vi "Teleop.vi"(10 "Match Info":T1={"Autonomous Elapsed Seconds"=0.0, "TeleOp Elapsed Seconds"=0.0, "Disabled Elapsed Seconds"=0.0, "Visited Autonomous"=FALSE, "Visited TeleOp"=FALSE, "Visited Disabled"=FALSE, "Autonomous Settings"={"Autonomous Style"=enum."Independent", "VI Refnum"=refnum}}, 11 "Call Context":T2) -> ()   [LabVIEW 2019]
doc: "This VI is called for each TeleOp packet received from the DS where the robot is not disabled. It is often used to read from the joysticks and update I/O or to update setpoints for timed control loops. It should complete and return within 20 milliseconds or it may miss DS packets."
uses:
  <vilib>/Rock Robotics/WPI/DriverStation/WPI_DriverStationDerivedRobotMode.ctl
  <vilib>/Rock Robotics/WPI/DriverStation/WPI_DriverStationMatch Info.ctl
  <vilib>/Rock Robotics/WPI/ThirdParty/JAS_Junk/TrajLib/Conv_Meters_Feet.vi
  <vilib>/Rock Robotics/WPI/ThirdParty/JAS_Junk/TrajLib/Conv_Radians_Deg.vi
  <vilib>/Rock Robotics/WPI/Utilities/WPI_GetSetVariantRefNum.vi
  <vilib>/Rock Robotics/Network Tables/NT Write Boolean Array.vi
  <vilib>/Rock Robotics/Network Tables/NT Write Numeric Array.vi
  <vilib>/Rock Robotics/WPI/Joystick/WPI_JoystickArcadeMapping.vi
  Robot Global Data.vi
  <vilib>/Rock Robotics/Network Tables/NT Read Boolean.vi
  <vilib>/Rock Robotics/WPI/ThirdParty/JAS_Junk/TrajLib/Trajectory_Library.lvlib
  <vilib>/Rock Robotics/Network Tables/NT Read Number.vi
panel:
  out "Sample Slider 0":dbl(slide) scale=0.0..5.0
  out "Sample Boolean 1":bool
  out "Sample Boolean 0":bool
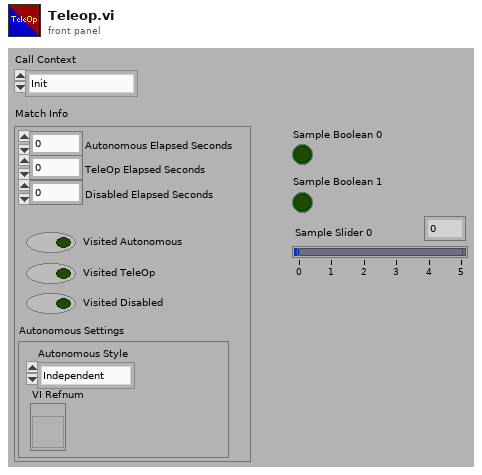
[diagram p1: front panel]
types:
  T1 = typedef "WPI_DriverStationMatch Info.ctl" = cluster{"Autonomous Elapsed Seconds":dbl, "TeleOp Elapsed Seconds":dbl, "Disabled Elapsed Seconds":dbl, "Visited Autonomous":bool, "Visited TeleOp":bool, "Visited Disabled":bool, "Autonomous Settings":cluster{"Autonomous Style":enum16{"Iterative", "Independent"}, "VI Refnum":refnum<vi>}}
  T2 = typedef "WPI_DriverStationDerivedRobotMode.ctl" = enum16{"Init", "Execute", "Stop"}
  T3 = typedef "WPI_JoystickDevRef.ctl" = cluster{"Device":T4}
  T4 = typedef "WPI_JoystickDeviceEnum.ctl" = enum16{"USB 0", "USB 1", "USB 2", "USB 3", "USB 4", "USB 5"}
  T5 = typedef "Trajectory_Library.lvlib/RAMSETE.ctl" = cluster{"B":dbl, "Zeta":dbl, "poseTolerance":T6, "poseError":T6, "Enabled":bool}
  T6 = typedef "Trajectory_Library.lvlib/POSE2D.ctl" = cluster{"TRANSLATION":T7, "ROTATION":T8}
  T7 = typedef "Trajectory_Library.lvlib/TRANSLATION2D.ctl" = cluster{"X":dbl, "Y":dbl}
  T8 = typedef "Trajectory_Library.lvlib/ROTATION2D.ctl" = cluster{"VALUE":dbl, "COS":dbl, "SIN":dbl}
  T9 = typedef "Trajectory_Library.lvlib/TRAJ_STATE.ctl" = cluster{"TimeSeconds":dbl, "Velocity":dbl, "Acceleration":dbl, "POSE":T6, "Curvature":dbl}
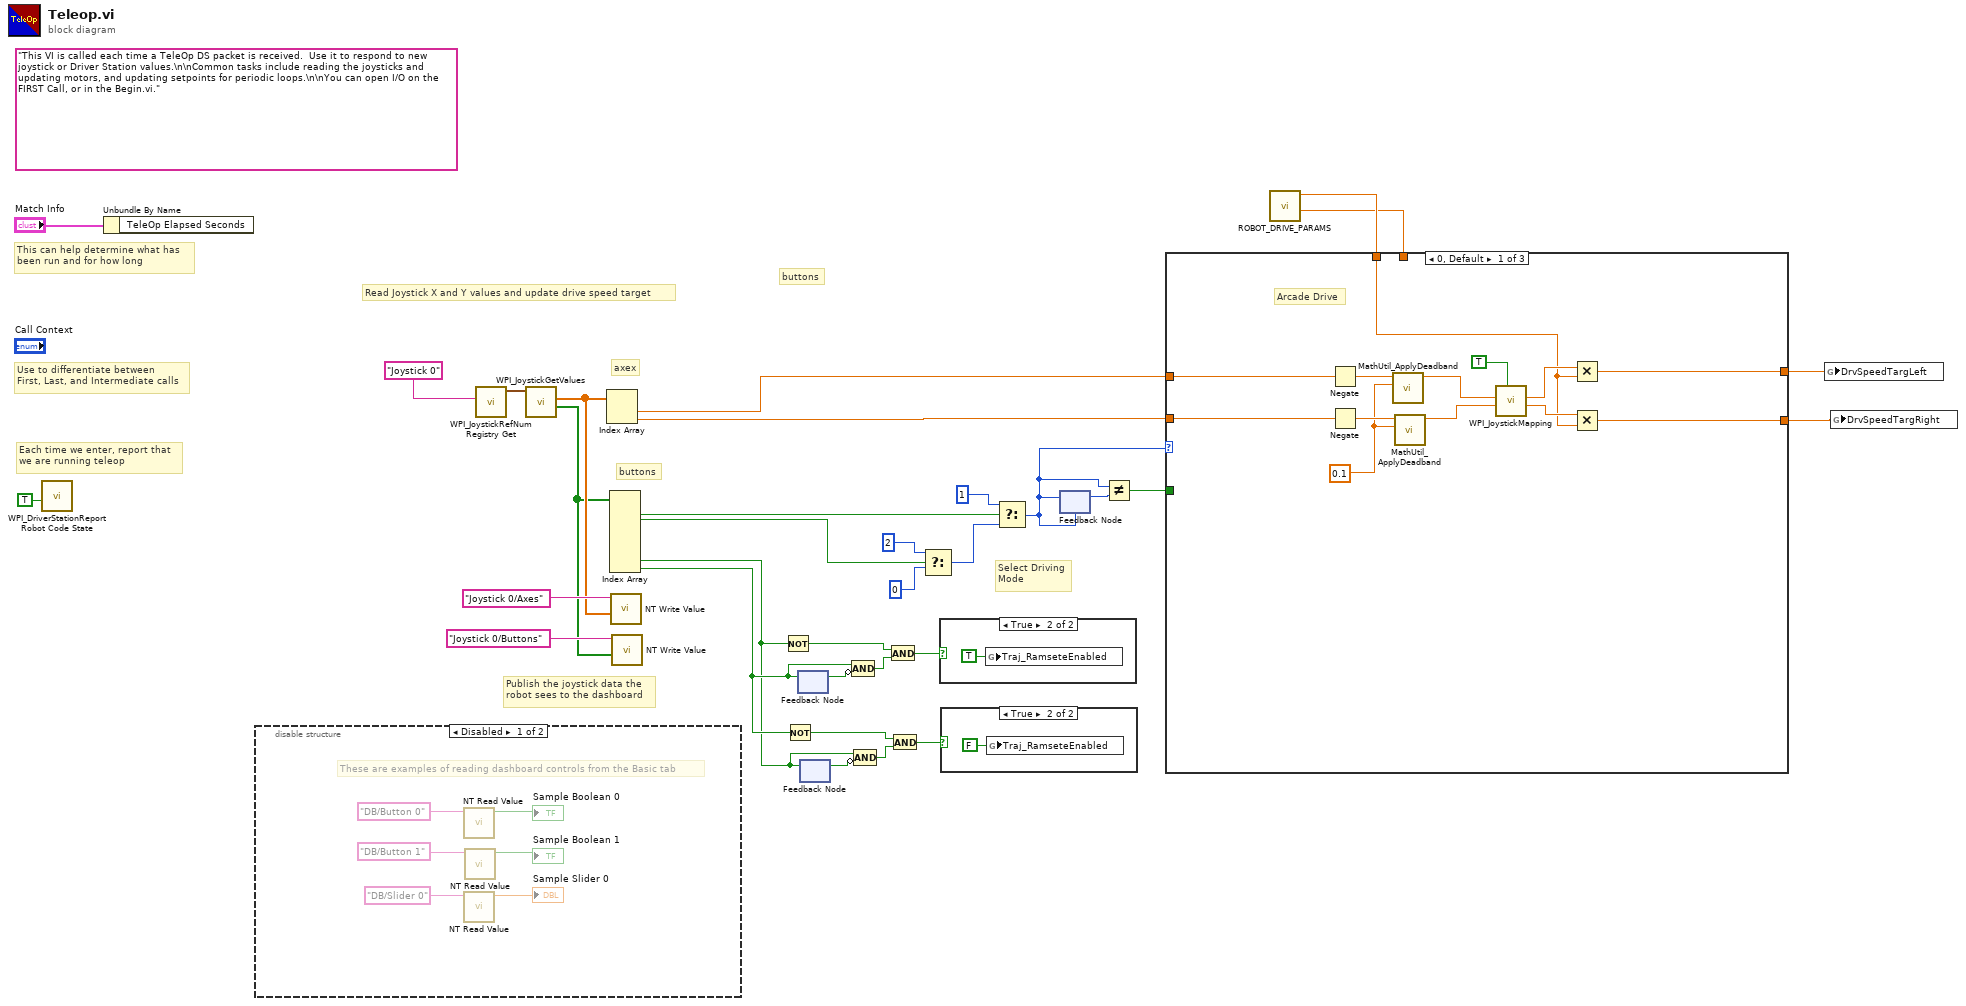
[diagram p0: block diagram]
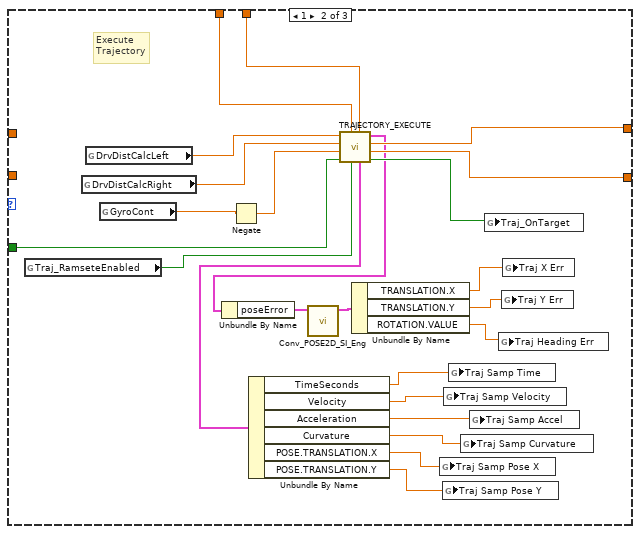
[diagram p4: hidden frame]
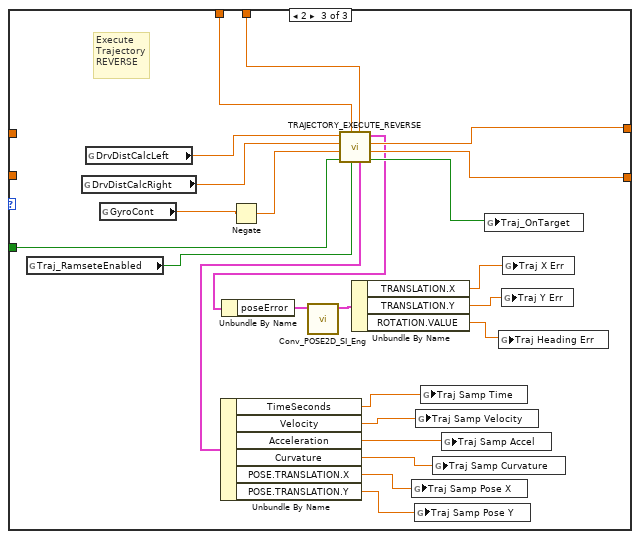
[diagram p5: hidden frame]
diagram:
  (unwired) "This VI is called each time a TeleOp DS packet is received.  Use it to respond to new joystick or Driver Station values.\n\nCommon tasks include reading the joysticks and updating motors, and updating setpoints for periodic loops.\n\nYou can open I/O on the FIRST Call, or in the Begin.vi."
  # "buttons"
  # "Select Driving\nMode"
  # "buttons"
  # "axex"
  # "Publish the joystick data the\nrobot sees to the dashboard"
  # "Each time we enter, report that\nwe are running teleop"
  # "Use to differentiate between\nFirst, Last, and Intermediate calls"
  # "This can help determine what has\nbeen run and for how long"
  # "Read Joystick X and Y values and update drive speed target"
  n1 = call <vilib>:"WPI_DriverStationReport Robot Code State.vi"("TeleOp"=TRUE ("Autonomous")) -> ()  [unwired: 10 in, 1 out]
  n2 = Unbundle By Name("Match Info") -> ()  [unwired: 1 out]
  n3 = disable-structure shown="Disabled" {
    frame Disabled {
      # "These are examples of reading dashboard controls from the Basic tab"
      n4 = call-poly <vilib>:"NT Read Value.vi"("Name"="DB/Button 0" ("refnum name")) -> ("Boolean"=→"Sample Boolean 0":bool)  [unwired: 9 in, 1 out]
      n5 = call-poly <vilib>:"NT Read Value.vi"("Name"="DB/Slider 0" ("refnum name")) -> ("Numeric"=→"Sample Slider 0":dbl)  [unwired: 9 in, 1 out]
      n6 = call-poly <vilib>:"NT Read Value.vi"("Name"="DB/Button 1" ("refnum name")) -> ("Boolean"=→"Sample Boolean 1":bool)  [unwired: 9 in, 1 out]
    }
    frame Enabled {
    }
  }
  n7 = call <vilib>:"WPI_JoystickRefNum Registry Get.vi"("refnum name"="Joystick 0") -> ("JoystickDevRef"=w31:T3)  [unwired: 1 in, 9 out]
  n8 = call <vilib>:"WPI_JoystickGetValues.vi"("JoystickDevRef"=w31) -> ("Buttons"=w21:bool[], "Axes"=w27:dbl[])  [unwired: 6 in, 3 out]
  n9 = Index Array(array=w27) -> (element #1=w26:dbl, element #2=w25:dbl)  [unwired: 2 in]
  n10 = Index Array(array=w21) -> (element #1=w19:bool, element #2=w12:bool, element #7=w1:bool, element #8=w2:bool)  [unwired: 8 in, 4 out]
  n11 = call-poly <vilib>:"NT Write Value.vi"("Numeric Array"=w27, "Name"="Joystick 0/Axes") -> ()  [unwired: 9 in, 1 out]
  n12 = call-poly <vilib>:"NT Write Value.vi"("Boolean Array"=w21, "Name"="Joystick 0/Buttons") -> ()  [unwired: 9 in, 1 out]
  n13 = Not(x=w1) -> (.not. x?=w8:bool)
  n14 = Not(x=w2) -> (.not. x?=w5:bool)
  n15 = feedback #1() -> (w10:bool)  [unwired: 1 in]
  n16 = feedback-in #1(w2) -> ()
  n17 = feedback #2() -> (w7:bool)  [unwired: 1 in]
  n18 = feedback-in #2(w1) -> ()
  n19 = Compound Arithmetic op=AND(w2, invert w10) -> (w9:bool)
  n20 = Compound Arithmetic op=AND(w1, invert w7) -> (w6:bool)
  n21 = And(x=w8, y=w9) -> (x .and. y?=w3:bool)
  n22 = And(x=w5, y=w6) -> (x .and. y?=w4:bool)
  n23 = Select(t=2, s=w12, f=0) -> (s? t:f=w13:i32)
  n24 = case shown="True" w3 {
    frame False {
    }
    frame True {
      n25 = global write "Robot Global Data.vi" "Traj_RamseteEnabled"(TRUE ("Traj_RamseteEnabled")) -> ()
    }
  }
  n26 = case shown="True" w4 {
    frame False {
    }
    frame True {
      n27 = global write "Robot Global Data.vi" "Traj_RamseteEnabled"(FALSE ("Traj_RamseteEnabled")) -> ()
    }
  }
  n28 = Select(t=1, s=w19, f=w13) -> (s? t:f=w17:i32)
  n29 = feedback-in #3(w17) -> ()
  n30 = feedback #3(w17) -> (w18:i32)
  n31 = Not Equal?(x=w17, y=w18) -> (x != y?=w16:bool)
  n32 = call "ROBOT_DRIVE_PARAMS.vi"() -> ("Effective Wheelbase Ft"=w11:dbl, "Max Speed Ft/Sec"=w22:dbl)  [unwired: 10 in]
  n33 = case shown="0, Default" w17 {
    tunnel: w26 -> [w53 _ _]
    tunnel: w25 -> [w52 _ _]
    tunnel: [w51 w72 w96] -> w24
    tunnel: [w50 w71 w95] -> w23
    tunnel: w22 -> [w47 w73 w97]
    tunnel: w16 -> [_ w78 w102]
    tunnel: w11 -> [_ w57 w81]
    frame 0, Default {
      w42 = 0.1 ("Deadband")
      # "Arcade Drive"
      n34 = Negate(x=w53) -> (-x=w45:dbl)
      n35 = Negate(x=w52) -> (-x=w44:dbl)
      n36 = call <vilib>:"MathUtil_ApplyDeadband.vi"("Deadband"=w42, "Value"=w45) -> ("Result"=w46:dbl)  [unwired: 9 in]
      n37 = call <vilib>:"MathUtil_ApplyDeadband.vi"("Deadband"=w42, "Value"=w44) -> ("Result"=w43:dbl)  [unwired: 9 in]
      n38 = call-poly <vilib>:"WPI_JoystickMapping.vi"("Square Inputs"=TRUE, "Y axis value"=w43, "X axis value"=w46) -> ("Right Motor Value"=w48:dbl, "Left Motor Value"=w49:dbl)  [unwired: 7 in]
      n39 = Multiply(x=w49, y=w47) -> (x*y=w51:dbl)
      n40 = Multiply(x=w48, y=w47) -> (x*y=w50:dbl)
    }
    frame 1 {
      # "Execute\nTrajectory"
      n41 = global read "Robot Global Data.vi" "Traj_RamseteEnabled"() -> (w55:bool)
      n42 = global read "Robot Global Data.vi" "DrvDistCalcRight"() -> (w75:dbl)
      n43 = global read "Robot Global Data.vi" "DrvDistCalcLeft"() -> (w76:dbl)
      n44 = global read "Robot Global Data.vi" "GyroCont"() -> (w77:dbl)
      n45 = Negate(x=w77) -> (-x=w74:dbl)
      n46 = call "TRAJECTORY_EXECUTE.vi"("Track Width FT"=w57, "RamseteEnable"=w55, "Max Speed\nFT/SEC"=w73, "Init"=w78, "Gyro Continous\n (inc counterclockwise)"=w74, "Right Distance"=w75, "Left Distance"=w76) -> ("AtReference"=w70:bool, "Right Speed Target"=w71:dbl, "Left Speed Target"=w72:dbl, "outRAMSETE (SI)"=w69:T5, "OutputTRAJ_STATE (SI)"=w56:T9)
      n47 = Unbundle By Name(w69) -> ("poseError"=w68:T6)
      n48 = Unbundle By Name(w56) -> ("TimeSeconds"=w63:dbl, "Velocity"=w62:dbl, "Acceleration"=w61:dbl, "Curvature"=w60:dbl, "POSE.TRANSLATION.X"=w59:dbl, "POSE.TRANSLATION.Y"=w58:dbl)
      n49 = call <vilib>:"Conv_POSE2D_SI_Eng.vi"("Err Pose in SI"=w68) -> ("Err Pose out ENG"=w67:T6)  [unwired: 10 in]
      n50 = Unbundle By Name(w67) -> ("TRANSLATION.X"=w66:dbl, "TRANSLATION.Y"=w65:dbl, "ROTATION.VALUE"=w64:dbl)
      n51 = global write "Robot Global Data.vi" "Traj Samp Pose X"(w59) -> ()
      n52 = global write "Robot Global Data.vi" "Traj Samp Pose Y"(w58) -> ()
      n53 = global write "Robot Global Data.vi" "Traj Samp Velocity"(w62) -> ()
      n54 = global write "Robot Global Data.vi" "Traj Samp Time"(w63) -> ()
      n55 = global write "Robot Global Data.vi" "Traj Samp Curvature"(w60) -> ()
      n56 = global write "Robot Global Data.vi" "Traj Samp Accel"(w61) -> ()
      n57 = global write "Robot Global Data.vi" "Traj_OnTarget"(w70) -> ()
      n58 = global write "Robot Global Data.vi" "Traj Heading Err"(w64) -> ()
      n59 = global write "Robot Global Data.vi" "Traj Y Err"(w65) -> ()
      n60 = global write "Robot Global Data.vi" "Traj X Err"(w66) -> ()
    }
    frame 2 {
      # "Execute\nTrajectory\nREVERSE"
      n61 = global read "Robot Global Data.vi" "Traj_RamseteEnabled"() -> (w79:bool)
      n62 = global read "Robot Global Data.vi" "DrvDistCalcRight"() -> (w99:dbl)
      n63 = global read "Robot Global Data.vi" "DrvDistCalcLeft"() -> (w100:dbl)
      n64 = global read "Robot Global Data.vi" "GyroCont"() -> (w101:dbl)
      n65 = Negate(x=w101) -> (-x=w98:dbl)
      n66 = call "TRAJECTORY_EXECUTE_REVERSE.vi"("Track Width FT"=w81, "RamseteEnable"=w79, "Max Speed\nFT/SEC"=w97, "Init"=w102, "Gyro Continous\n (inc counterclockwise)"=w98, "Right Distance"=w99, "Left Distance"=w100) -> ("AtReference"=w94:bool, "Right Speed Target"=w95:dbl, "Left Speed Target"=w96:dbl, "outRAMSETE (SI)"=w93:T5, "OutputTRAJ_STATE (SI)"=w80:T9)
      n67 = Unbundle By Name(w80) -> ("TimeSeconds"=w87:dbl, "Velocity"=w86:dbl, "Acceleration"=w85:dbl, "Curvature"=w84:dbl, "POSE.TRANSLATION.X"=w83:dbl, "POSE.TRANSLATION.Y"=w82:dbl)
      n68 = Unbundle By Name(w93) -> ("poseError"=w92:T6)
      n69 = call <vilib>:"Conv_POSE2D_SI_Eng.vi"("Err Pose in SI"=w92) -> ("Err Pose out ENG"=w91:T6)  [unwired: 10 in]
      n70 = Unbundle By Name(w91) -> ("TRANSLATION.X"=w90:dbl, "TRANSLATION.Y"=w89:dbl, "ROTATION.VALUE"=w88:dbl)
      n71 = global write "Robot Global Data.vi" "Traj Samp Pose X"(w83) -> ()
      n72 = global write "Robot Global Data.vi" "Traj Samp Pose Y"(w82) -> ()
      n73 = global write "Robot Global Data.vi" "Traj Samp Velocity"(w86) -> ()
      n74 = global write "Robot Global Data.vi" "Traj Samp Time"(w87) -> ()
      n75 = global write "Robot Global Data.vi" "Traj Samp Curvature"(w84) -> ()
      n76 = global write "Robot Global Data.vi" "Traj Samp Accel"(w85) -> ()
      n77 = global write "Robot Global Data.vi" "Traj_OnTarget"(w94) -> ()
      n78 = global write "Robot Global Data.vi" "Traj Heading Err"(w88) -> ()
      n79 = global write "Robot Global Data.vi" "Traj Y Err"(w89) -> ()
      n80 = global write "Robot Global Data.vi" "Traj X Err"(w90) -> ()
    }
  }
  n81 = global write "Robot Global Data.vi" "DrvSpeedTargLeft"(w24) -> ()
  n82 = global write "Robot Global Data.vi" "DrvSpeedTargRight"(w23) -> ()
